vi "update_dust_type.vi"(8 "error in (no error)":errorcluster, 11 "ID Dust Type":i32) -> (0 "error out":errorcluster)   [LabVIEW 2013]
doc: "Menu: Allows the user to edit a given dust type or create a new dust type."
uses:
  <vilib>/Utility/miscctls.llb/LVPointTypeDef.ctl
  <vilib>/Utility/error.llb/DialogType.ctl
  <userlib>/_OpenG.lib/string/string.llb/To Proper Case (String Array)__ogtk.vi
  <vilib>/addons/database/_DB Variant To Data/Database Variant To Data.xnode
panel:
  out "Update Query in Standard Format":string
  in  "Cancel":bool caption="Update Dust Entry"
  in  "New Dust Entry":bool caption="Update Dust Entry"
  in  "Update Dust Entry":bool
  in  "Dust Type":T1
  out "Query in Standard Format":string
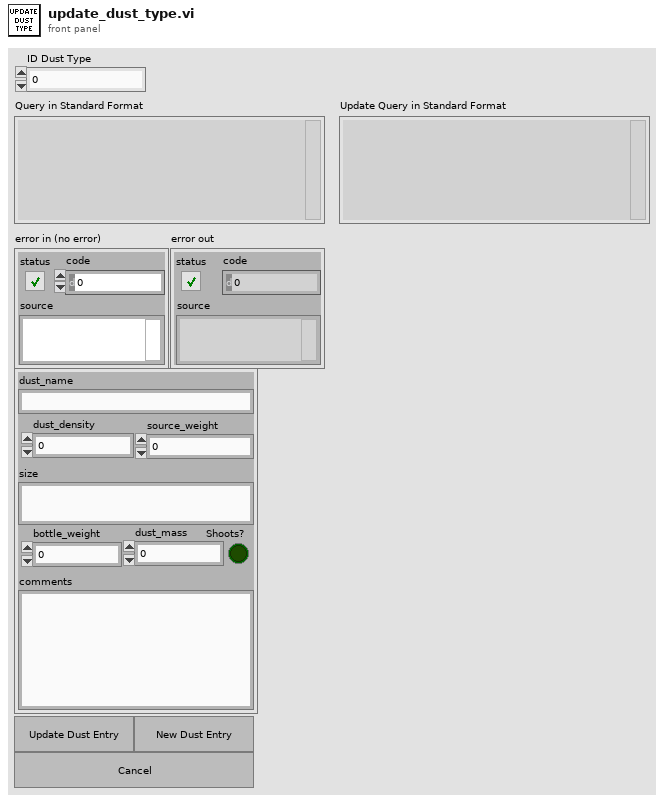
[diagram p1: front panel]
types:
  T1 = cluster{"id_dust_type":i32, "dust_name":string, "dust_type":i32, "batch_no":i32, "dust_density":dbl, "source_weight":dbl, "size":string, "bottle_weight":dbl, "dust_mass":dbl, "comments":string, "Shoots?":bool}
  T2 = typedef "LVPointTypeDef.ctl" = cluster{"Horizontal":i16, "Vertical":i16}
  T3 = typedef "DialogType.ctl" = u16
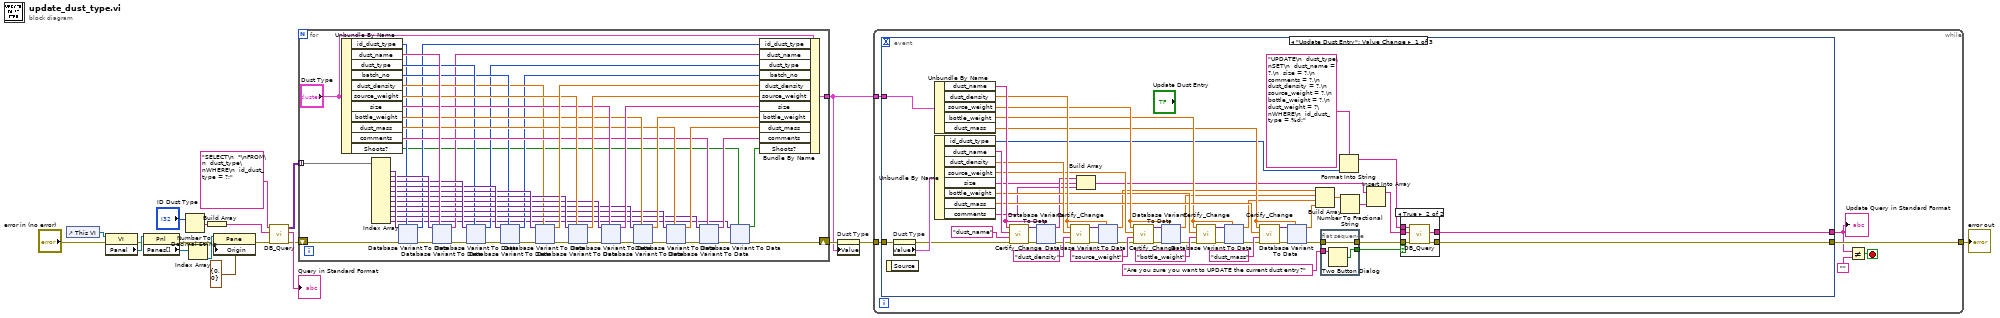
[diagram p0: block diagram]
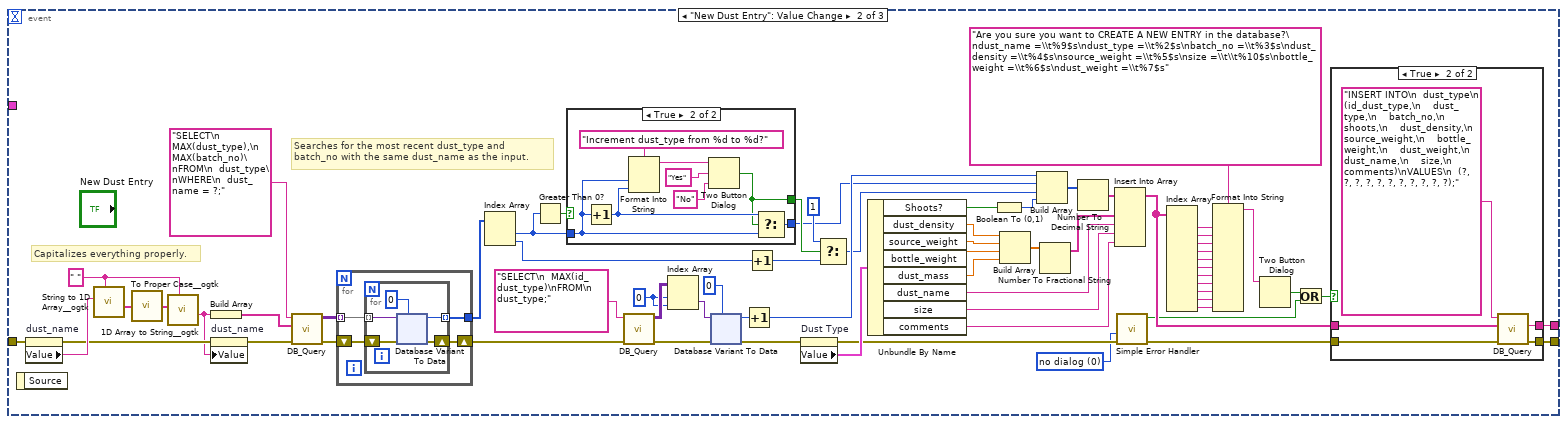
[diagram p3: hidden frame]
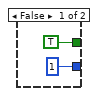
[diagram p5: hidden frame]
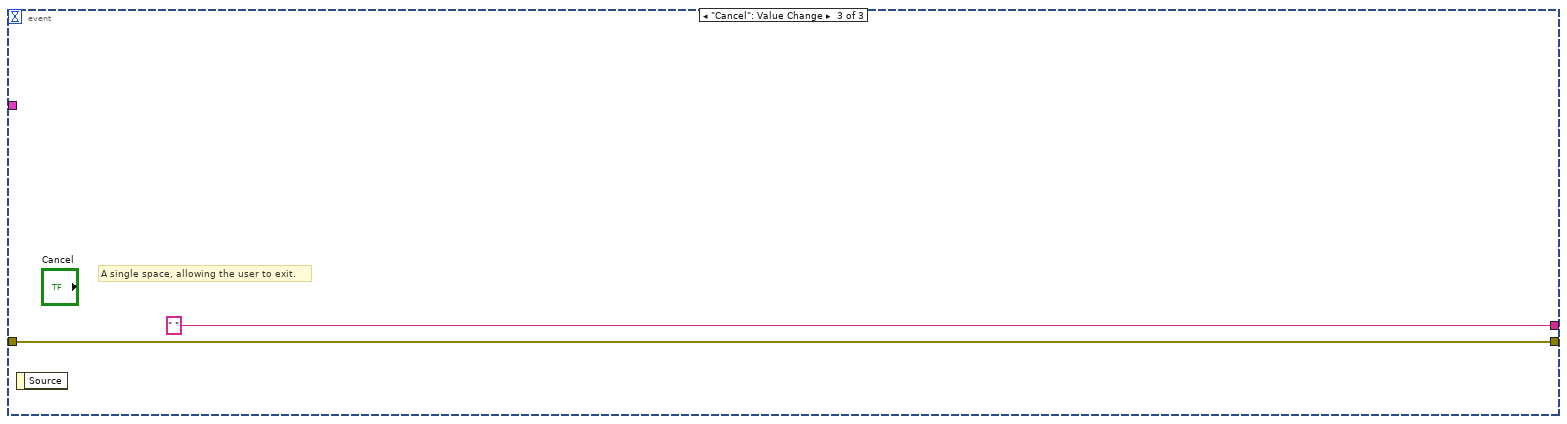
[diagram p6: hidden frame]
diagram:
  n1 = control-ref of="This VI"() -> (w10:refnum<vi>)
  n2 = property class="VI"(reference=w10, error in="error in (no error)") -> (error out=w11:errorcluster, "Panel"=w12:refnum<vi>)  [unwired: 1 out]
  n3 = property class="Pnl"(reference=w12, error in=w11) -> (error out=w13:errorcluster, "Panes[]"=w14:refnum<vi>[])  [unwired: 1 out]
  n4 = Number To Decimal String(number="ID Dust Type") -> (decimal integer string=w6:string)  [unwired: 1 in]
  n5 = Index Array(array=w14) -> (element=w15:refnum<vi>)  [unwired: 1 in]
  n6 = Build Array(w6) -> (w5:string[])
  n7 = property class="Pane"(reference=w15, error in=w13, "Origin"=T2 {"Horizontal"=0, "Vertical"=0}) -> (error out=w8:errorcluster)  [unwired: 1 out]
  n8 = call "DB_Query.vi"("error in (no error)"=w8, "Parameters"=w5, "Parameterized Query"="SELECT\n  *\nFROM\n  dust_type\nWHERE\n  id_dust_type = ?;") -> ("error out"=w19:errorcluster, "Query in Standard Format"=→"Query in Standard Format":string, "Results"=w18:variant[][])  [unwired: 6 in]
  n9 = for {
    shift-right: [w21] -> w17
    shift-left: w19 -> [w66]
    tunnel: [w67] -> w1
    tunnel: w18 -> [w27] mode=indexing
    n10 = Unbundle By Name("Dust Type") -> ("id_dust_type"=w29:i32, "dust_name"=w62:string, "dust_type"=w34:i32, "batch_no"=w33:i32, "dust_density"=w32:dbl, "source_weight"=w53:dbl, "size"=w48:string, "bottle_weight"=w45:dbl, "dust_mass"=w40:dbl, "comments"=w36:string, "Shoots?"=w23:bool)
    n11 = Index Array(array=w27) -> (element #1=w65:variant, element #2=w63:variant, element #3=w60:variant, element #4=w58:variant, element #5=w56:variant, element #6=w52:variant, element #7=w49:variant, element #8=w44:variant, element #9=w41:variant, element #10=w37:variant, element #11=w24:variant)  [unwired: 11 in]
    n12 = xnode "Database Variant To Data"("database variant"=w65, "error in (no error)"=w66, "type"=w29) -> ("data"=w28:i32, "error out"=w64:errorcluster)
    n13 = xnode "Database Variant To Data"("database variant"=w63, "error in (no error)"=w64, "type"=w62) -> ("data"=w26:string, "error out"=w61:errorcluster)
    n14 = xnode "Database Variant To Data"("database variant"=w60, "error in (no error)"=w61, "type"=w34) -> ("data"=w30:i32, "error out"=w59:errorcluster)
    n15 = xnode "Database Variant To Data"("database variant"=w58, "error in (no error)"=w59, "type"=w33) -> ("data"=w31:i32, "error out"=w57:errorcluster)
    n16 = xnode "Database Variant To Data"("database variant"=w56, "error in (no error)"=w57, "type"=w32) -> ("data"=w55:dbl, "error out"=w54:errorcluster)
    n17 = xnode "Database Variant To Data"("database variant"=w52, "error in (no error)"=w54, "type"=w53) -> ("data"=w50:dbl, "error out"=w51:errorcluster)
    n18 = xnode "Database Variant To Data"("database variant"=w49, "error in (no error)"=w51, "type"=w48) -> ("data"=w47:string, "error out"=w46:errorcluster)
    n19 = xnode "Database Variant To Data"("database variant"=w44, "error in (no error)"=w46, "type"=w45) -> ("data"=w43:dbl, "error out"=w42:errorcluster)
    n20 = xnode "Database Variant To Data"("database variant"=w41, "error in (no error)"=w42, "type"=w40) -> ("data"=w39:dbl, "error out"=w38:errorcluster)
    n21 = xnode "Database Variant To Data"("database variant"=w37, "error in (no error)"=w38, "type"=w36) -> ("data"=w35:string, "error out"=w25:errorcluster)
    n22 = xnode "Database Variant To Data"("database variant"=w24, "error in (no error)"=w25, "type"=w23) -> ("data"=w22:bool, "error out"=w21:errorcluster)
    n23 = Bundle By Name(cluster="Dust Type", "id_dust_type"=w28, "dust_name"=w26, "dust_type"=w30, "batch_no"=w31, "dust_density"=w55, "source_weight"=w50, "size"=w47, "bottle_weight"=w43, "dust_mass"=w39, "comments"=w35, "Shoots?"=w22) -> (w67:T1)
  }
  n24 = property on="Dust Type" class="Clust (strict)"(error in=w17, "Value"=w1) -> (error out=w3:errorcluster)  [unwired: 1 in, 1 out]
  n25 = while {
    tunnel: w3 -> [w426]
    tunnel: [w425] -> w2
    tunnel: w1 -> [w424]
    stop <- w422 stop-if-true
    n26 = event shown="[0] \"Update Dust Entry\": Value Change" {
      selector: _ -> [_ _ _]
      dyn-events: _ -> [_ _ _]
      timeout: _ -> [_ _ _]
      tunnel: w426 -> [w475 w713 w805]
      tunnel: [w479 w715 w805] -> w425
      tunnel: [w478 w714 " "] -> w421
      tunnel: w424 -> [w470 _ _]
      event "Update Dust Entry": Value Change {
        n27 = event-data() -> ()  [unwired: 1 in, 1 out]
        n28 = property on="Dust Type" class="Clust (strict)"(error in=w475) -> (error out=w473:errorcluster, "Value"=w474:T1)  [unwired: 1 in, 1 out]
        n29 = Unbundle By Name(w470) -> ("dust_name"=w469:string, "dust_density"=w463:dbl, "source_weight"=w453:dbl, "bottle_weight"=w446:dbl, "dust_mass"=w445:dbl)
        n30 = Unbundle By Name(w474) -> ("id_dust_type"=w427:i32, "dust_name"=w471:string, "dust_density"=w464:dbl, "source_weight"=w458:dbl, "size"=w438:string, "bottle_weight"=w448:dbl, "dust_mass"=w447:dbl, "comments"=w437:string)
        n31 = call "Certify_Change.vi"("error in (no error)"=w473, "Variable Name"="dust_name", "New Value"=w471, "Default Value"=w469) -> ("error out"=w477:errorcluster, "Value Out"=w476:variant)  [unwired: 6 in]
        n32 = xnode "Database Variant To Data"("database variant"=w476, "error in (no error)"=w477, "type"=w469) -> ("data"=w439:string, "error out"=w465:errorcluster)
        n33 = call "Certify_Change.vi"("error in (no error)"=w465, "Variable Name"="dust_density", "New Value"=w464, "Default Value"=w463) -> ("error out"=w466:errorcluster, "Value Out"=w467:variant)  [unwired: 6 in]
        n34 = Build Array(w439, w438, w437) -> (w436:string[])
        n35 = xnode "Database Variant To Data"("database variant"=w467, "error in (no error)"=w466, "type"=w463) -> ("data"=w444:dbl, "error out"=w459:errorcluster)
        n36 = call "Certify_Change.vi"("error in (no error)"=w459, "Variable Name"="source_weight", "New Value"=w458, "Default Value"=w453) -> ("error out"=w462:errorcluster, "Value Out"=w461:variant)  [unwired: 6 in]
        n37 = xnode "Database Variant To Data"("database variant"=w461, "error in (no error)"=w462, "type"=w453) -> ("data"=w443:dbl, "error out"=w454:errorcluster)
        n38 = call "Certify_Change.vi"("error in (no error)"=w454, "Variable Name"="bottle_weight", "New Value"=w448, "Default Value"=w446) -> ("error out"=w455:errorcluster, "Value Out"=w456:variant)  [unwired: 6 in]
        n39 = xnode "Database Variant To Data"("database variant"=w456, "error in (no error)"=w455, "type"=w446) -> ("data"=w442:dbl, "error out"=w449:errorcluster)
        n40 = call "Certify_Change.vi"("error in (no error)"=w449, "Variable Name"="dust_mass", "New Value"=w447, "Default Value"=w445) -> ("error out"=w452:errorcluster, "Value Out"=w451:variant)  [unwired: 6 in]
        n41 = xnode "Database Variant To Data"("database variant"=w451, "error in (no error)"=w452, "type"=w445) -> ("data"=w441:dbl, "error out"=w432:errorcluster)
        n42 = Build Array(w444, w443, w442, w441) -> (w440:dbl[])
        n43 = flat-sequence {
          tunnel: [w482] -> w433
          tunnel: w432 -> [w482]
          tunnel: [w481] -> w431
          tunnel: "Are you sure you want to UPDATE the current dust entry?" ("message") -> [w480]
          frame #0 {
            n44 = Two Button Dialog(message=w480) -> (T button?=w481:bool)  [unwired: 2 in]
          }
        }
        n45 = Format Into String(format string="UPDATE\n  dust_type\nSET\n  dust_name = ?,\n  size = ?,\n  comments = ?,\n  dust_density = ?,\n  source_weight = ?,\n  bottle_weight = ?,\n  dust_weight = ?\nWHERE\n  id_dust_type = %d;" ("Parameterized Query"), w427) -> (resulting string=w429:string)  [unwired: 2 in, 1 out]
        n46 = Number To Fractional String(number=w440) -> (F-format string=w435:string[])  [unwired: 3 in]
        n47 = Insert Into Array(array=w436, new element=w435) -> (w434:string[])  [unwired: 1 in]
        n48 = case shown="True" w431 {
          tunnel: [w483 w488] -> w479
          tunnel: [_ w487] -> w478
          tunnel: w429 -> [_ w486]
          tunnel: w434 -> [_ w485]
          tunnel: w433 -> [w483 w484]
          frame False {
          }
          frame True {
            n49 = call "DB_Query.vi"("error in (no error)"=w484, "Parameters"=w485, "Parameterized Query"=w486) -> ("error out"=w488:errorcluster, "Query in Standard Format"=w487:string)  [unwired: 6 in, 1 out]
          }
        }
      }
      event "New Dust Entry": Value Change {
        w671 = T3 0 items=["no dialog", "OK message", "continue or stop message", "OK message + warnings", "continue/stop + warnings"] ("type of dialog (OK msg:1)")
        w697 = 0 ("index (row)")
        w710 = " " ("delimiter (Tab)")
        # "Searches for the most recent dust_type and\nbatch_no with the same dust_name as the input."
        # "Capitalizes everything properly."
        n50 = event-data() -> ()  [unwired: 1 in, 1 out]
        n51 = property on="dust_name" class="Str"(error in=w713) -> (error out=w693:errorcluster, "Value"=w708:string)  [unwired: 1 in, 1 out]
        n52 = call <userlib>:"String to 1D Array__ogtk.vi"("delimiter (Tab)"=w710, "string"=w708) -> ("Array of Strings"=w711:string[])  [unwired: 9 in]
        n53 = call-poly <userlib>:"To Proper Case__ogtk.vi"("strings"=w711) -> ("proper case strings"=w709:string[])  [unwired: 4 in]
        n54 = call <userlib>:"1D Array to String__ogtk.vi"("delimiter (Tab)"=w710, "Array of Strings"=w709) -> ("delimited string"=w691:string)  [unwired: 9 in]
        n55 = Build Array(w691) -> (w707:string[])
        n56 = property on="dust_name" class="Str"(error in=w693, "Value"=w691) -> (error out=w692:errorcluster)  [unwired: 1 in, 1 out]
        n57 = call "DB_Query.vi"("error in (no error)"=w692, "Parameters"=w707, "Parameterized Query"="SELECT\n  MAX(dust_type),\n  MAX(batch_no)\nFROM\n  dust_type\nWHERE\n  dust_name = ?;") -> ("error out"=w705:errorcluster, "Results"=w706:variant[][])  [unwired: 6 in, 1 out]
        n58 = for {
          tunnel: w706 -> [w766] mode=indexing
          shift-right: [w765] -> w689
          shift-left: w705 -> [w767]
          tunnel: [w764] -> w704
          n59 = for {
            shift-right: [w771] -> w765
            shift-left: w767 -> [w772]
            tunnel: w766 -> [w770] mode=indexing
            tunnel: [w768] -> w764 mode=indexing
            n60 = xnode "Database Variant To Data"("database variant"=w770, "error in (no error)"=w772, "type"=0) -> ("data"=w768:i32, "error out"=w771:errorcluster)
          }
        }
        n61 = Index Array(array=w704) -> (element #1=w688:i32, element #2=w701:i32)  [unwired: 2 in]
        n62 = Greater Than 0?(x=w688) -> (x > 0?=w703:bool)
        n63 = case shown="True" w703 {
          tunnel: w688 -> [_ w760]
          tunnel: [TRUE ("T button?") w759] -> w702
          tunnel: [1 ("data") w758] -> w650
          frame False {
          }
          frame True {
            n64 = Increment(x=w760) -> (x+1=w761:i32)
            n65 = Format Into String(format string="Increment dust_type from %d to %d?" ("message"), w760, w761) -> (resulting string=w763:string)  [unwired: 2 in, 1 out]
            n66 = Two Button Dialog(message=w763, 1:"No" ("F button name (\"Cancel\")"), 2:"Yes" ("T button name (\"OK\")")) -> (T button?=w759:bool)
            n67 = Select(t=w761, s=w759, f=w760) -> (s? t:f=w758:i32)
          }
        }
        n68 = call "DB_Query.vi"("error in (no error)"=w689, "Parameterized Query"="SELECT\n  MAX(id_dust_type)\nFROM\n  dust_type;") -> ("error out"=w699:errorcluster, "Results"=w698:variant[][])  [unwired: 7 in, 1 out]
        n69 = Index Array(array=w698, index (row)=w697, index (col)=w697) -> (element=w696:variant)
        n70 = xnode "Database Variant To Data"("database variant"=w696, "error in (no error)"=w699, "type"=0) -> ("data"=w694:i32, "error out"=w687:errorcluster)
        n71 = Increment(x=w694) -> (x+1=w690:i32)
        n72 = Increment(x=w701) -> (x+1=w649:i32)
        n73 = property on="Dust Type" class="Clust (strict)"(error in=w687) -> (error out=w673:errorcluster, "Value"=w683:T1)  [unwired: 1 in, 1 out]
        n74 = Select(t=1, s=w702, f=w649) -> (s? t:f=w685:i32)
        n75 = Unbundle By Name(w683) -> ("Shoots?"=w652:bool, "dust_density"=w651:dbl, "source_weight"=w679:dbl, "bottle_weight"=w678:dbl, "dust_mass"=w677:dbl, "dust_name"=w676:string, "size"=w675:string, "comments"=w674:string)
        n76 = Boolean To (0,1)(Boolean=w652) -> (0, 1=w670:i16)
        n77 = Build Array(w651, w679, w678, w677) -> (w680:dbl[])
        n78 = Build Array(w690, w650, w685, w670) -> (w684:i32[])
        n79 = Number To Fractional String(number=w680) -> (F-format string=w681:string[])  [unwired: 3 in]
        n80 = Number To Decimal String(number=w684) -> (decimal integer string=w682:string[])  [unwired: 1 in]
        n81 = Insert Into Array(array=w682, new element #1=w681, new element #2=w676, new element #3=w675, new element #4=w674) -> (w669:string[])  [unwired: 1 in]
        n82 = call <vilib>:"Simple Error Handler.vi"("type of dialog (OK msg:1)"=w671, "error in (no error)"=w673) -> ("error?"=w655:bool, "error out"=w672:errorcluster)  [unwired: 3 in, 3 out]
        n83 = Index Array(array=w669) -> (element #1=w658:string, element #2=w659:string, element #3=w660:string, element #4=w661:string, element #5=w662:string, element #6=w663:string, element #7=w664:string, element #8=w665:string, element #9=w666:string, element #10=w667:string, element #11=w668:string)  [unwired: 11 in]
        n84 = Format Into String(format string="Are you sure you want to CREATE A NEW ENTRY in the database?\ndust_name =\\t%9$s\ndust_type =\\t%2$s\nbatch_no =\\t%3$s\ndust_density =\\t%4$s\nsource_weight =\\t%5$s\nsize =\\t\\t%10$s\nbottle_weight =\\t%6$s\ndust_weight =\\t%7$s", w658, w659, w660, w661, w662, w663, w664, w665, w666, w667, w668) -> (resulting string=w654:string)  [unwired: 2 in, 1 out]
        n85 = Two Button Dialog(message=w654) -> (T button?=w657:bool)  [unwired: 2 in]
        n86 = Or(x=w657, y=w655) -> (x .or. y?=w656:bool)
        n87 = case shown="True" w656 {
          tunnel: [w716 w721] -> w715
          tunnel: [_ w720] -> w714
          tunnel: w672 -> [w716 w718]
          tunnel: w669 -> [_ w717]
          frame False {
          }
          frame True {
            n88 = call "DB_Query.vi"("error in (no error)"=w718, "Parameters"=w717, "Parameterized Query"="INSERT INTO\n  dust_type\n    (id_dust_type,\n    dust_type,\n    batch_no,\n    shoots,\n    dust_density,\n    source_weight,\n    bottle_weight,\n    dust_weight,\n    dust_name,\n    size,\n    comments)\nVALUES\n  (?, ?, ?, ?, ?, ?, ?, ?, ?, ?, ?);") -> ("error out"=w721:errorcluster, "Query in Standard Format"=w720:string)  [unwired: 6 in, 1 out]
          }
        }
      }
      event "Cancel": Value Change {
        # "A single space, allowing the user to exit."
        n89 = event-data() -> ()  [unwired: 1 in, 1 out]
      }
    }
    "Update Query in Standard Format" <- w421
    n90 = Not Equal?(x=w421, y="") -> (x != y?=w422:bool)
  }
  "error out" <- w2
